vi "PSAE_VCH_VCH List.vi"(8 "Error In (no error)":errorcluster) -> (0 "Error Out":errorcluster, 3 "VCHList":T1)   [LabVIEW 2016]
uses:
  VCH/Private/Ctrls/PSVCH_All Channels.ctl
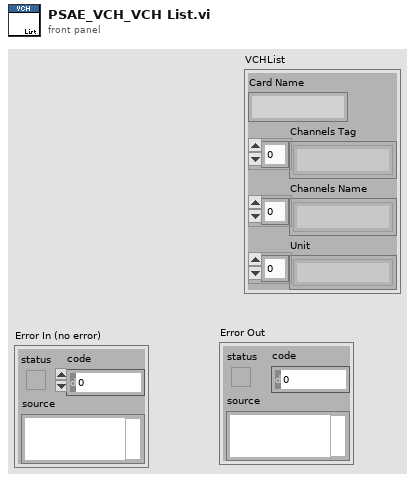
[diagram p1: front panel]
types:
  T1 = typedef "PSVCH_All Channels.ctl" = cluster{"Card Name":string, "Channels Tag":string[], "Channels Name":string[], "Unit":string[]}
  T2 = typedef "PSVCH_VCH Info.ctl" = cluster{"Tag":string[], "Tag String":string[], "Name":string[], "Enable":bool[], "Formula":string[], "Unit":string[], "Save":bool[], "Time":i64[]}
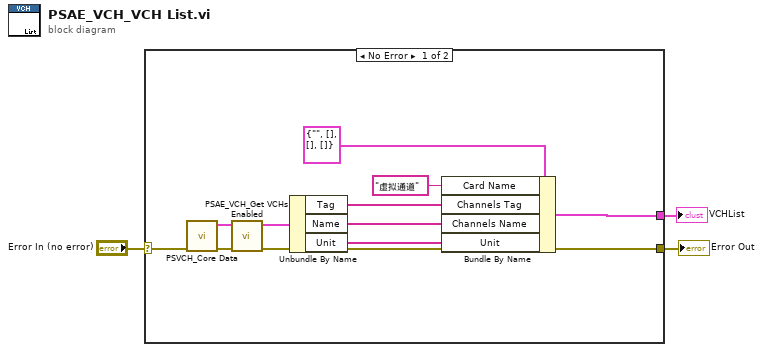
[diagram p0: block diagram]
diagram:
  n1 = case shown="No Error" "Error In (no error)" {
    selector: "Error In (no error)" -> [w14 w15]
    tunnel: [w6 w15] -> w2
    tunnel: [w5 _] -> w1
    frame No Error {
      n2 = call "PSVCH_Core Data.vi"("Error In (no error)"=w14) -> ("Error Out"=w13:errorcluster, "VCH Out"=w12:T2)  [unwired: 9 in]
      n3 = call "PSAE_VCH_Get VCHs Enabled.vi"("Error In (no error)"=w13, "VCH"=w12) -> ("Error Out"=w6:errorcluster, "VCH"=w11:T2)  [unwired: 8 in]
      n4 = Unbundle By Name(w11) -> ("Tag"=w8:string[], "Name"=w7:string[], "Unit"=w4:string[])
      n5 = Bundle By Name(cluster=T1 {"Card Name"="", "Channels Tag"=[], "Channels Name"=[], "Unit"=[]} ("DAQ2ANA"), "Card Name"="虚拟通道", "Channels Tag"=w8, "Channels Name"=w7, "Unit"=w4) -> (w5:T1)
    }
    frame Error {
    }
  }
  "Error Out" <- w2
  "VCHList" <- w1
